vi "Create A New File.vi"(7 "Path in":path, 8 "Blocking requirements":cluster{"Value":dbl, " Number":i32}[](array[cluster]), 9 "Subject #":string, 10 "Filename":string, 11 "Mode":string) -> (3 "Path out":path)   [LabVIEW 2013]
uses:
  <vilib>/Utility/file.llb/Write To Spreadsheet File (string).vi
panel:
  in  "Case Constant\n(See Context Help)":bool
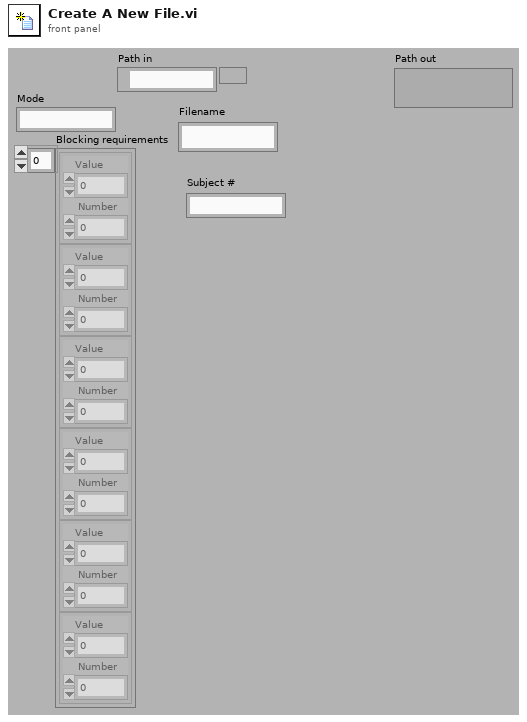
[diagram p1: front panel]
types:
  T1 = enum16{"open", "open or create", "create or replace", "create", "open (read only)"}
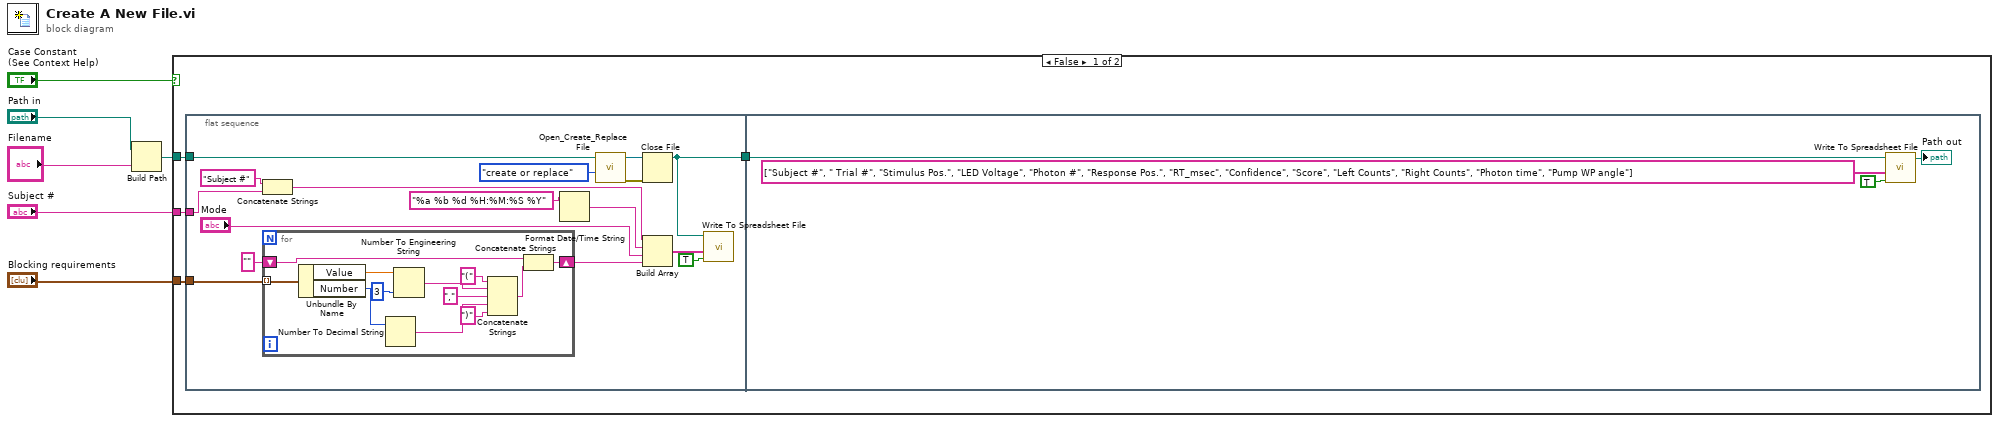
[diagram p0: block diagram]
diagram:
  n1 = Build Path(base path="Path in", name or relative path="Filename") -> (appended path=w6:path)
  n2 = case shown="False" "Case Constant\n(See Context Help)" {
    tunnel: w6 -> [w10 _]
    tunnel: "Subject #" -> [w8 _]
    tunnel: "Blocking requirements" -> [w7 _]
    frame False {
      n3 = flat-sequence {
        tunnel: w10 -> [w18]
        tunnel: [w21] -> w9
        tunnel: w8 -> [w17]
        tunnel: w7 -> [w15]
        tunnel: w9 -> [w41]
        frame #0 {
          n4 = Concatenate Strings("Subject #", w17) -> (w19:string)
          n5 = for {
            tunnel: w15 -> [w38] mode=indexing
            shift-right: [w29] -> w13
            shift-left: "" -> [w27]
            n6 = Unbundle By Name(w38) -> ("Value"=w36:dbl, "Number"=w32:i32)
            n7 = Number To Decimal String(number=w32) -> (decimal integer string=w31:string)  [unwired: 1 in]
            n8 = Number To Engineering String(2:i16 3 ("precision (6)"), 4:w36) -> (0:w34:string)  [unwired: 2 in]
            n9 = Concatenate Strings("(" ("string"), w34, "," ("string"), w31, ")" ("string")) -> (w28:string)
            n10 = Concatenate Strings(w27, w28) -> (w29:string)
          }
          n11 = Format Date/Time String(time format string (%c)="%a %b %d %H:%M:%S %Y") -> (date/time string=w12:string)  [unwired: 2 in]
          n12 = call <vilib>:"Open_Create_Replace File.vi"("function (open:0)"=T1."create or replace", "file path"=w18) -> ("error out"=w24:errorcluster, "refnum"=w23:refnum<file>)  [unwired: 6 in, 2 out]
          n13 = Close File(refnum=w23, error in=w24) -> (path=w21:path)  [unwired: 1 out]
          n14 = Build Array(w19, w12, "Mode", w13) -> (w26:string[])
          n15 = call-poly <vilib>:"Write To Spreadsheet File.vi"("append to file? (new file:F)"=TRUE, "1D data"=w26, "file path (dialog if empty)"=w21) -> ()  [unwired: 5 in, 1 out]
        }
        frame #1 {
          n16 = call-poly <vilib>:"Write To Spreadsheet File.vi"("append to file? (new file:F)"=TRUE, "1D data"=string[] ["Subject #", " Trial #", "Stimulus Pos.", "LED Voltage", "Photon #", "Response Pos.", "RT_msec", "Confidence", "Score", "Left Counts", "Right Counts", "Photon time", "Pump WP angle"], "file path (dialog if empty)"=w41) -> ("new file path (Not A Path if cancelled)"=→"Path out":path)  [unwired: 5 in]
        }
      }
    }
    frame True {
    }
  }
